vi "VI de controle.vi"() -> ()   [LabVIEW 2019]
panel:
  out "objective function":string
  in  "Tab Control":enum32{"Control panel", "Debug panel"}(tab)
  in  "Table Control":string[][](table)=[["fraise", "120", "10", "20", "30", "20", "0"], ["radis", "230", "20", "21", "10", "10", "0"], ["roquette", "150", "42", "26", "40", "20", "0"], ["laitue", "400", "35", "50", "52", "23", "0"], ["piment", "100", "51", "50", "20", "15", "0"], ["épinard", "170", "21", "12", "40", "10", "0"], ["basilic", "80", "12", "10", "10", "50", "0"]]
  in  "show system state":i32=1
  in  "time base":i32
  out "résultat":string
  out "données matlab":string
  in  "error in":errorcluster
  out "error out":errorcluster
  out "standard output":string
  out "standard error":string
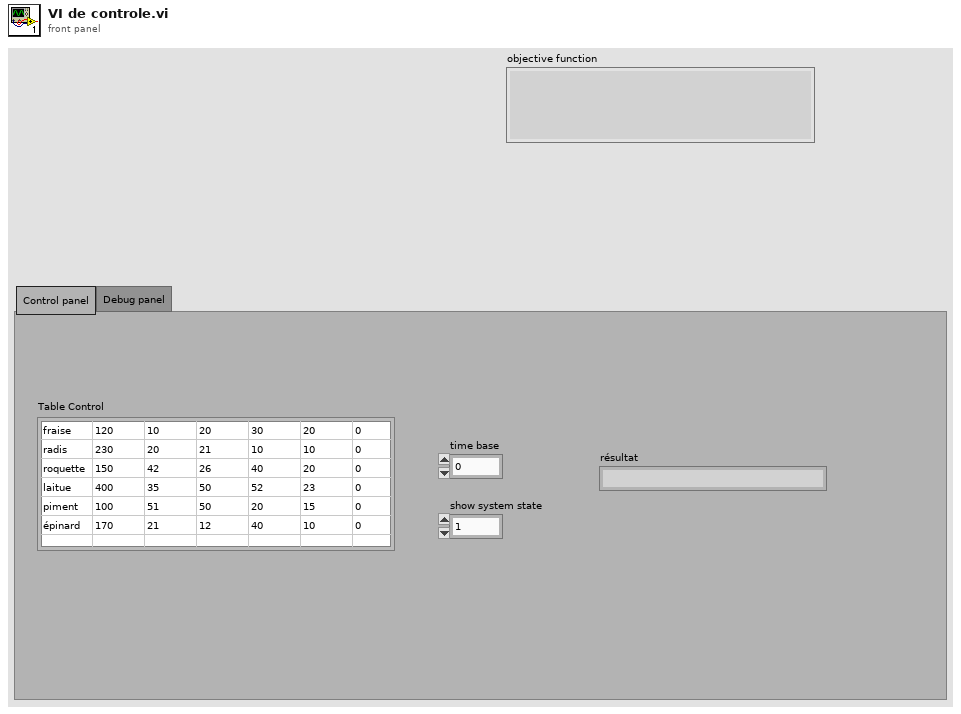
[diagram p1: front panel]
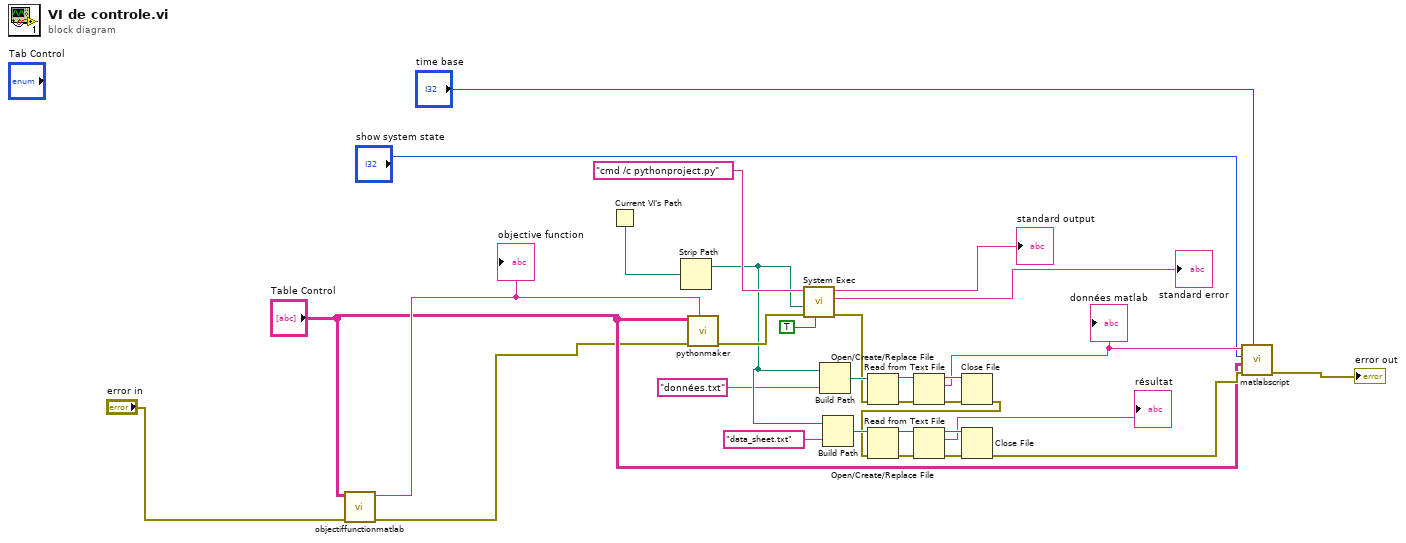
[diagram p0: block diagram]
diagram:
  n1 = call "objectiffunctionmatlab.vi"("error in (no error)"="error in", "Table Control"="Table Control") -> ("error out"=w1:errorcluster, "objective function"=w4:string)  [unwired: 8 in]
  "objective function" <- w4
  n2 = Current VI's Path() -> (path=w31:path)
  n3 = Strip Path(path=w31) -> (stripped path=w19:path)  [unwired: 1 out]
  n4 = call "pythonmaker.vi"("objective"=w4, "error in"=w1, "Table Control"="Table Control") -> ("error out"=w28:errorcluster)  [unwired: 8 in]
  n5 = call <vilib>:"System Exec.vi"("run minimized? (F)"=TRUE, "error in (no error)"=w28, "working directory"=w19, "command line"="cmd /c pythonproject.py") -> ("error out"=w13:errorcluster, "standard error"=→"standard error":string, "standard output"=→"standard output":string)  [unwired: 4 in, 1 out]
  n6 = Build Path(base path=w19, name or relative path="données.txt") -> (appended path=w21:path)
  n7 = Build Path(base path=w19, name or relative path="data_sheet.txt") -> (appended path=w20:path)
  n8 = Open/Create/Replace File(file path (use dialog)=w21, error in=w13) -> (refnum out=w18:refnum<file>, error out=w27:errorcluster)  [unwired: 4 in, 1 out]
  n9 = Read from Text File(file (use dialog)=w18, error in=w27) -> (refnum out=w25:refnum<file>, text=w11:string, error out=w26:errorcluster)  [unwired: 2 in, 1 out]
  "données matlab" <- w11
  n10 = Close File(refnum=w25, error in=w26) -> (error out=w12:errorcluster)  [unwired: 1 out]
  n11 = Open/Create/Replace File(file path (use dialog)=w20, error in=w12) -> (refnum out=w17:refnum<file>, error out=w24:errorcluster)  [unwired: 4 in, 1 out]
  n12 = Read from Text File(file (use dialog)=w17, error in=w24) -> (refnum out=w22:refnum<file>, text=→"résultat":string, error out=w23:errorcluster)  [unwired: 2 in, 1 out]
  n13 = Close File(refnum=w22, error in=w23) -> (error out=w10:errorcluster)  [unwired: 1 out]
  n14 = call "matlabscript.vi"("base de temps"="time base", "error in (no error)"=w10, "Table Control"="Table Control", "show system state"="show system state", "solver data"=w11) -> ("error out"=→"error out":errorcluster)  [unwired: 6 in]
